vi "Dialog - Configure Threading.vi"(6 "rxPacket?":bool, 7 "error in (no error)":errorcluster, 9 "threadOptions in":T2 {"pclDecimation" max=16 step=1; "loopPeriod" max=16 step=1; "targetPriority" min=-2 max=16 step=1; "targetProcessor" min=-2 max=16 step=1}, 10 "Packet Ref in":T1 format="%.0x") -> (0 "error out":errorcluster, 2 "threadOptions out":T2 {"pclDecimation" max=16 step=1; "loopPeriod" max=16 step=1; "targetPriority" min=-2 max=16 step=1; "targetProcessor" min=-2 max=16 step=1}, 3 "Packet Ref out":T1 format="%.0x")   [LabVIEW 2016, in "UDP-Custom-Device System Explorer.lvlib"]
uses:
  UDP-Custom-Device System Explorer.lvlib
  Types/Threading/Thread Sync Reference.ctl
  Types/Threading/Thread Configuration.ctl
  <vilib>/NI Veristand/Custom Device API/Custom Device Item Ref.ctl
  <vilib>/NI VeriStand/Custom Device API/Custom Device API.lvlib
panel:
  in  "threadSync":T3 caption="Synchronization"
  in  "pclDecimation":u16=1 caption="PCL Decimation" min=1 step=1
  in  "loopPeriod":u32=1 caption="Loop Period (us)" min=1 step=1
  in  "defaultPriority":bool
  in  "targetPriority":i16=1 caption="Priority" min=1 step=1
  in  "defaultProcessor":bool
  in  "targetProcessor":i8 caption="Target Processor" min=-2 max=16 step=1
  in  "Cancel":bool
  in  "OK":bool
  # "Select Packet Threading Options"
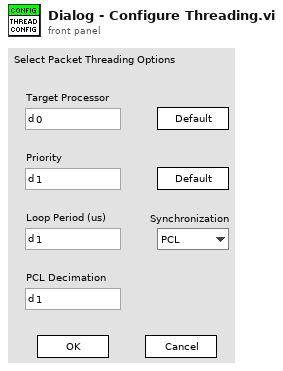
[diagram p1: front panel]
types:
  T1 = typedef "Custom Device API.lvlib/Custom Device Item Ref.ctl" = u64
  T2 = typedef "UDP-Custom-Device System Explorer.lvlib/Thread Configuration.ctl" = cluster{"targetProcessor":i8, "targetPriority":i16, "Synchronization":T3, "loopPeriod":u32, "pclDecimation":u16}
  T3 = typedef "UDP-Custom-Device System Explorer.lvlib/Thread Sync Reference.ctl" = enum16{"PCL", "Async"}
  T4 = enum8{"Enabled", "Disabled", "Disabled and Grayed Out"}
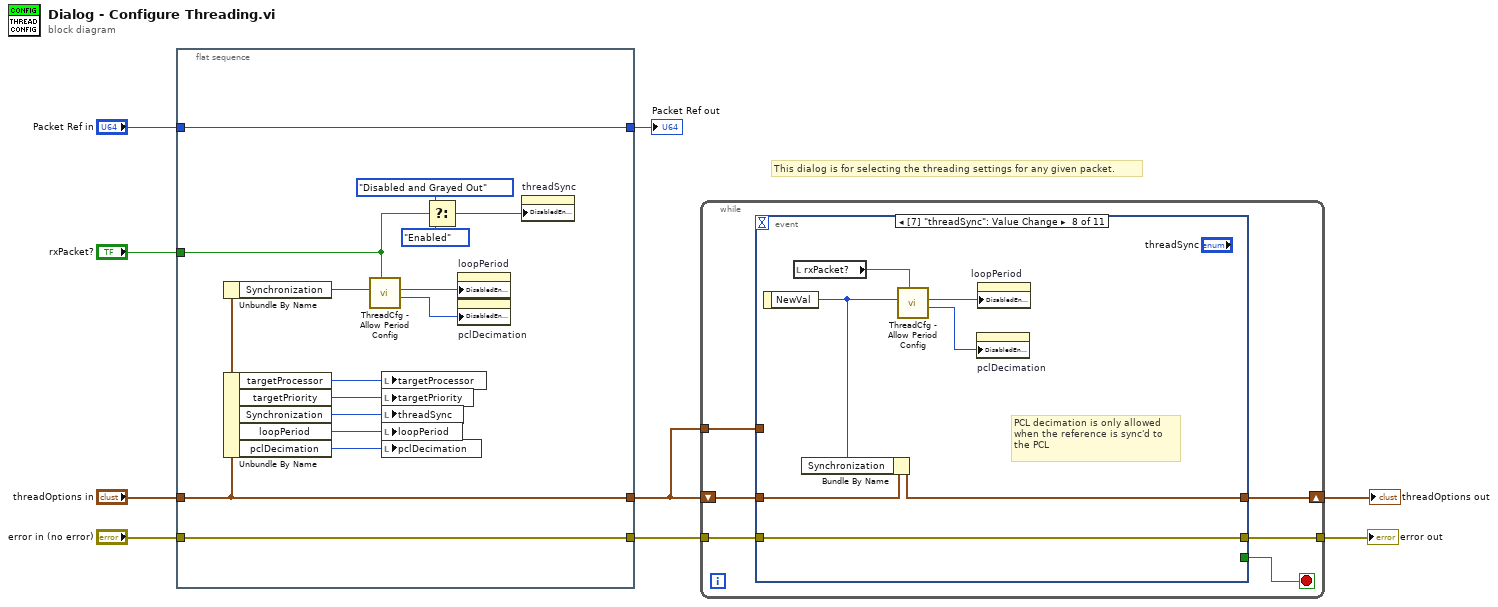
[diagram p0: block diagram]
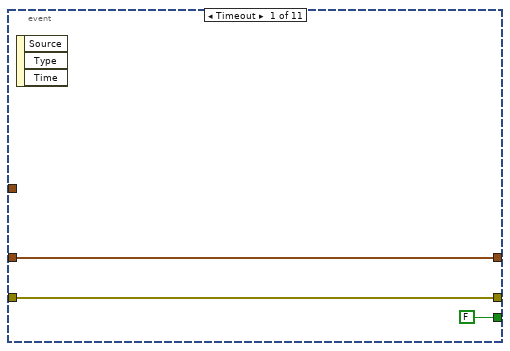
[diagram p2: hidden frame]
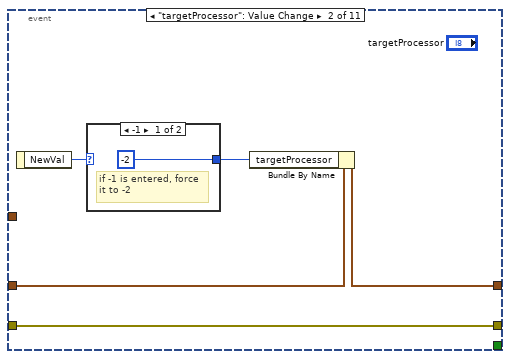
[diagram p3: hidden frame]
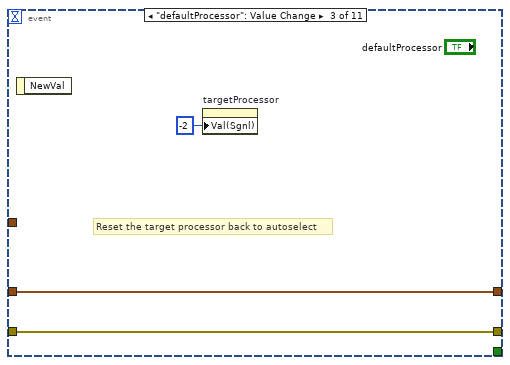
[diagram p5: hidden frame]
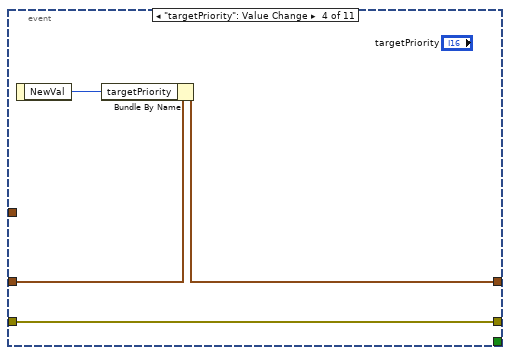
[diagram p6: hidden frame]
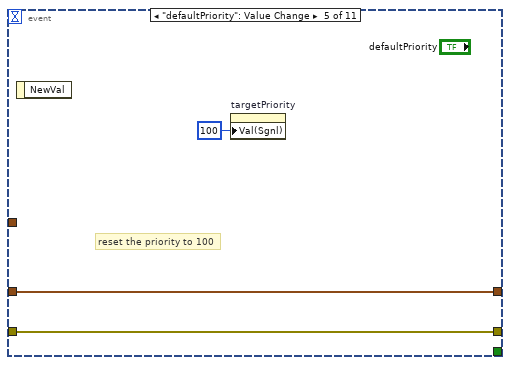
[diagram p7: hidden frame]
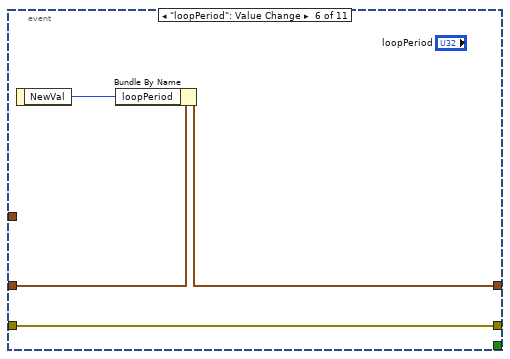
[diagram p8: hidden frame]
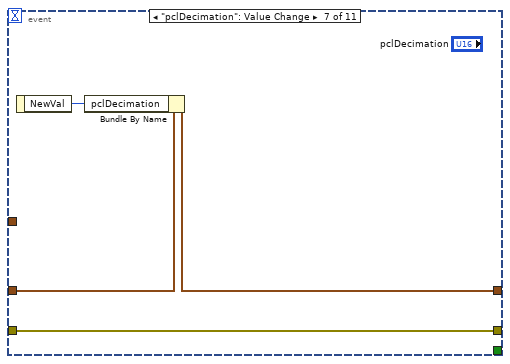
[diagram p9: hidden frame]
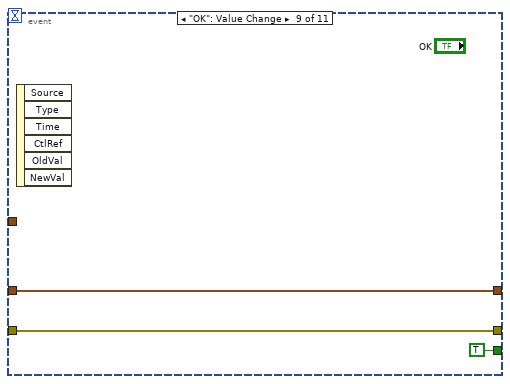
[diagram p10: hidden frame]
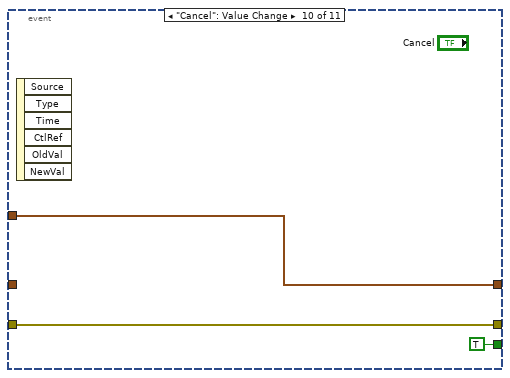
[diagram p11: hidden frame]
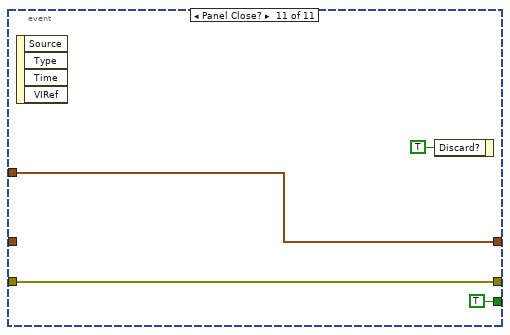
[diagram p12: hidden frame]
diagram:
  # "This dialog is for selecting the threading settings for any given packet."
  n1 = flat-sequence {
    tunnel: "error in (no error)" -> [w24]
    tunnel: [w24] -> w7
    tunnel: "threadOptions in" -> [w18]
    tunnel: [w18] -> w6
    tunnel: "rxPacket?" -> [w10]
    tunnel: [w14] -> w2
    tunnel: "Packet Ref in" -> [w14]
    frame #0 {
      n2 = Unbundle By Name(w18) -> ("Synchronization"=w17:T3)
      n3 = Unbundle By Name(w18) -> ("targetProcessor"=w19:i8, "targetPriority"=w20:i16, "Synchronization"=w21:T3, "loopPeriod"=w22:u32, "pclDecimation"=w23:u16)
      n4 = call "ThreadCfg - Allow Period Config.vi"("rxPacket?"=w10, "threadPeriodRef"=w17) -> ("pclDecimationState"=w15:T4, "loopPeriodState"=w16:T4)  [unwired: 8 in]
      n5 = local write "targetProcessor"(w19) -> ()
      n6 = local write "targetPriority"(w20) -> ()
      n7 = local write "threadSync"(w21) -> ()
      n8 = local write "loopPeriod"(w22) -> ()
      n9 = local write "pclDecimation"(w23) -> ()
      n10 = Select(t=T4."Disabled and Grayed Out" ("Disabled"), s=w10, f=T4."Enabled" ("Disabled")) -> (s? t:f=w11:T4)
      n11 = property on="loopPeriod" class="DigNum (strict)"("DisabledEnum"=w16) -> ()  [unwired: 2 in, 2 out]
      n12 = property on="pclDecimation" class="DigNum (strict)"("DisabledEnum"=w15) -> ()  [unwired: 2 in, 2 out]
      n13 = property on="threadSync" class="Enum (strict)"("DisabledEnum"=w11) -> ()  [unwired: 2 in, 2 out]
    }
  }
  n14 = while {
    tunnel: w7 -> [w28]
    shift-right: [w25] -> w4
    shift-left: w6 -> [w29]
    tunnel: w6 -> [w30]
    tunnel: [w26] -> w5
    stop <- w27 stop-if-true
    n15 = event shown="[7] \"threadSync\": Value Change" {
      selector: _ -> [_ _ _ _ _ _ _ _ _ _ _]
      dyn-events: _ -> [_ _ _ _ _ _ _ _ _ _ _]
      timeout: _ -> [_ _ _ _ _ _ _ _ _ _ _]
      tunnel: w30 -> [_ _ _ _ _ _ _ _ _ w70 w74]
      tunnel: w29 -> [w31 w37 w42 w45 w49 w53 w57 w64 w67 _ _]
      tunnel: w28 -> [w32 w38 w43 w47 w50 w54 w58 w65 w68 w71 w75]
      tunnel: [FALSE _ _ _ _ _ _ _ TRUE TRUE TRUE] -> w27
      tunnel: [w32 w38 w43 w47 w50 w54 w58 w65 w68 w71 w75] -> w26
      tunnel: [w31 w36 w42 w44 w49 w52 w56 w63 w67 w70 w74] -> w25
      event Timeout {
        n16 = event-data() -> ()  [unwired: 1 in, 3 out]
      }
      event "targetProcessor": Value Change {
        n17 = event-data() -> ("NewVal"=w35:i8)  [unwired: 1 in]
        n18 = case shown="-1" w35 {
          selector: w35 -> [_ w40]
          tunnel: [i8 -2 w40] -> w34
          frame -1 {
            # "if -1 is entered, force\nit to -2"
          }
          frame Default {
          }
        }
        n19 = Bundle By Name(cluster=w37, "targetProcessor"=w34) -> (w36:T2)
      }
      event "defaultProcessor": Value Change {
        # "Reset the target processor back to autoselect"
        n20 = event-data() -> ()  [unwired: 1 in, 1 out]
        n21 = property on="targetProcessor" class="DigNum (strict)"("Val(Sgnl)"=i8 -2 ("Value (Signaling)")) -> ()  [unwired: 2 in, 2 out]
      }
      event "targetPriority": Value Change {
        n22 = event-data() -> ("NewVal"=w46:i16)  [unwired: 1 in]
        n23 = Bundle By Name(cluster=w45, "targetPriority"=w46) -> (w44:T2)
      }
      event "defaultPriority": Value Change {
        # "reset the priority to 100"
        n24 = event-data() -> ()  [unwired: 1 in, 1 out]
        n25 = property on="targetPriority" class="DigNum (strict)"("Val(Sgnl)"=i16 100 ("Value (Signaling)")) -> ()  [unwired: 2 in, 2 out]
      }
      event "loopPeriod": Value Change {
        n26 = event-data() -> ("NewVal"=w51:u32)  [unwired: 1 in]
        n27 = Bundle By Name(cluster=w53, "loopPeriod"=w51) -> (w52:T2)
      }
      event "pclDecimation": Value Change {
        n28 = event-data() -> ("NewVal"=w55:u16)  [unwired: 1 in]
        n29 = Bundle By Name(cluster=w57, "pclDecimation"=w55) -> (w56:T2)
      }
      event Value Change {
        # "PCL decimation is only allowed\nwhen the reference is sync'd to\nthe PCL"
        n30 = event-data() -> ("NewVal"=w61:T3)  [unwired: 1 in]
        n31 = local read "rxPacket?"() -> (w62:bool)
        n32 = Bundle By Name(cluster=w64, "Synchronization"=w61) -> (w63:T2)
        n33 = call "ThreadCfg - Allow Period Config.vi"("rxPacket?"=w62, "threadPeriodRef"=w61) -> ("pclDecimationState"=w59:T4, "loopPeriodState"=w60:T4)  [unwired: 8 in]
        n34 = property on="pclDecimation" class="DigNum (strict)"("DisabledEnum"=w59) -> ()  [unwired: 2 in, 2 out]
        n35 = property on="loopPeriod" class="DigNum (strict)"("DisabledEnum"=w60) -> ()  [unwired: 2 in, 2 out]
      }
      event "OK": Value Change {
        n36 = event-data() -> ()  [unwired: 1 in, 6 out]
      }
      event "Cancel": Value Change {
        n37 = event-data() -> ()  [unwired: 1 in, 6 out]
      }
      event Panel Close? {
        n38 = event-data() -> ()  [unwired: 1 in, 4 out]
        n39 = event-data("Discard?"=TRUE) -> ()  [unwired: 1 in, 1 out]
      }
    }
  }
  "error out" <- w5
  "threadOptions out" <- w4
  "Packet Ref out" <- w2
